vi "Config Wiring.vi"(0 "VISA resource name":refnum<visa-resource-name>, 5 "Wiring A (0: P1W2)":u16(ring) items=["P1W2", "P1W3", "P3W3", "P3W4", "V3A3"], 7 "Wiring B (0: P1W2)":u16(ring) items=["P1W2", "P1W3", "P3W3", "P3W4", "V3A3", "NONE"], 11 "error in (no error)":errorcluster) -> (4 "VISA resource name out":refnum<visa-resource-name>, 15 "error out":errorcluster)   [LabVIEW 2013, in "Yokogawa.lvlib" / "Yokogawa PZ4000.lvlib"]
doc: "This VI sends the Wiring Configure command to the PZ4000 series."
uses:
  Yokogawa PZ4000.lvlib
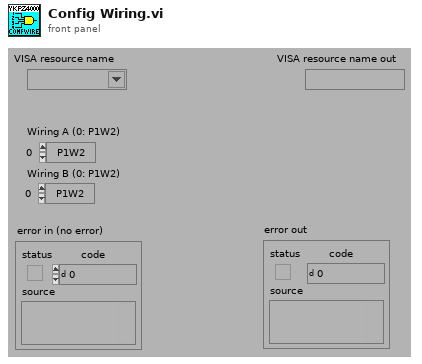
[diagram p1: front panel]
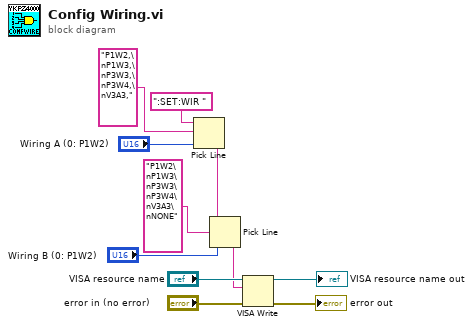
[diagram p0: block diagram]
diagram:
  n1 = Pick Line(string ("")=":SET:WIR ", multi-line string="P1W2,\nP1W3,\nP3W3,\nP3W4,\nV3A3,", line index="Wiring A (0: P1W2)") -> (output string=w3:string)
  n2 = Pick Line(string ("")=w3, multi-line string="P1W2\nP1W3\nP3W3\nP3W4\nV3A3\nNONE", line index="Wiring B (0: P1W2)") -> (output string=w2:string)
  n3 = VISA Write(VISA resource name="VISA resource name", write buffer=w2, error in (no error)="error in (no error)") -> (VISA resource name out=→"VISA resource name out":refnum<visa-resource-name>, error out=→"error out":errorcluster)  [unwired: 1 out]
